vi "VLC-IP_Play_Media_to_PictureBox.vi"(5 ".NET PictureBox":refnum<k24>(container), 8 "error in (no error)":errorcluster, 11 "VLC-IP":T1) -> (0 "error out":errorcluster, 3 "VLC-IP out":T1)   [LabVIEW 2016]
uses:
  System.Windows.Forms
  VLC-IP.ctl
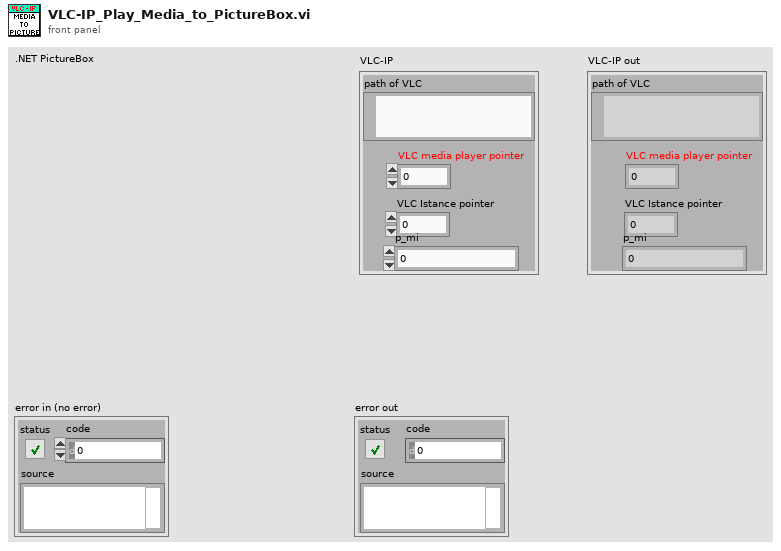
[diagram p1: front panel]
types:
  T1 = typedef "VLC-IP.ctl" = cluster{"path of VLC":path, "VLC media player pointer":i32, "VLC Istance pointer":i32, "p_mi":i32}
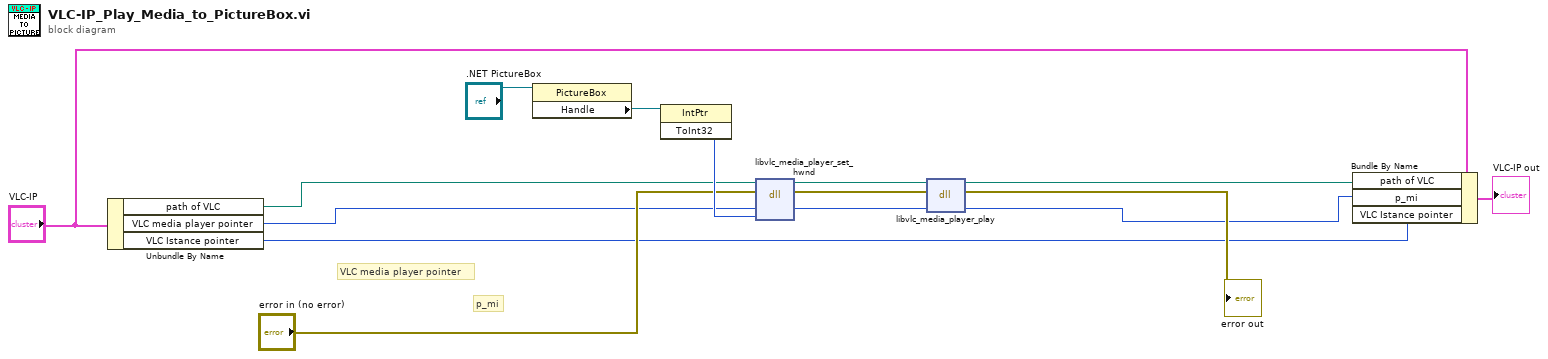
[diagram p0: block diagram]
diagram:
  # "VLC media player pointer"
  # "p_mi"
  n1 = Unbundle By Name("VLC-IP") -> ("path of VLC"=w7:path, "VLC media player pointer"=w6:i32, "VLC Istance pointer"=w2:i32)
  n2 = property class="PictureBox"(reference=".NET PictureBox") -> ("Handle"=w14:refnum<k24>)  [unwired: 1 in, 2 out]
  n3 = invoke class="IntPtr" method="ToInt32"(reference=w14) -> ("ToInt32"=w15:i32)  [unwired: 2 in, 2 out]
  n4 = dll-call lib="C:/Program Files (x86)/VideoLAN/VLC/libvlc.dll" fn="libvlc_media_player_set_hwnd"(path in=w7, error in="error in (no error)", "p_mi"=w6, "drawable"=w15) -> (path out=w9:path, error out=w11:errorcluster, "p_mi"=w10:i32)  [unwired: 3 in]
  n5 = dll-call lib="C:/Program Files (x86)/VideoLAN/VLC/libvlc.dll" fn="libvlc_media_player_play"(path in=w9, error in=w11, "p_mi"=w10) -> (path out=w4:path, error out=→"error out":errorcluster, "p_mi"=w3:i32)  [unwired: 2 in]
  n6 = Bundle By Name(cluster="VLC-IP", "path of VLC"=w4, "p_mi"=w3, "VLC Istance pointer"=w2) -> (→"VLC-IP out":T1)
